vi "Set Node Action.vi"(8 "error in (no error)":errorcluster, 9 "action-only":bool, 10 "nodeIndex":i32, 11 "FSM in":refnum<class "FSM.Graph.lvclass">) -> (0 "error out":errorcluster, 3 "FSM out":refnum<class "FSM.Graph.lvclass">)   [LabVIEW 2015, in "FSM.Graph.lvclass"]
uses:
  FSM.Graph.lvclass
  FSM.Graph.lvclass/FSM.Graph.ctl
  FSM.Node/Shape.ctl
  FSM.Node/FSM.Node.lvclass/FSM.Node.ctl
  FSM.Node/Write Shape.vi
  FSM.Node/FSM.Node.lvclass
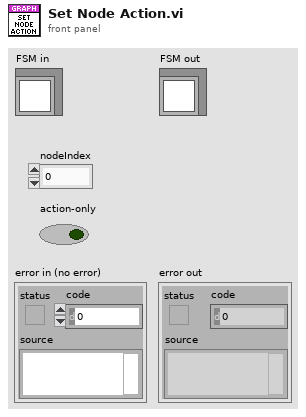
[diagram p1: front panel]
types:
  T1 = typedef "FSM.Node.lvclass/Shape.ctl" = enum16{"Default", "Start", "Action", "End"}
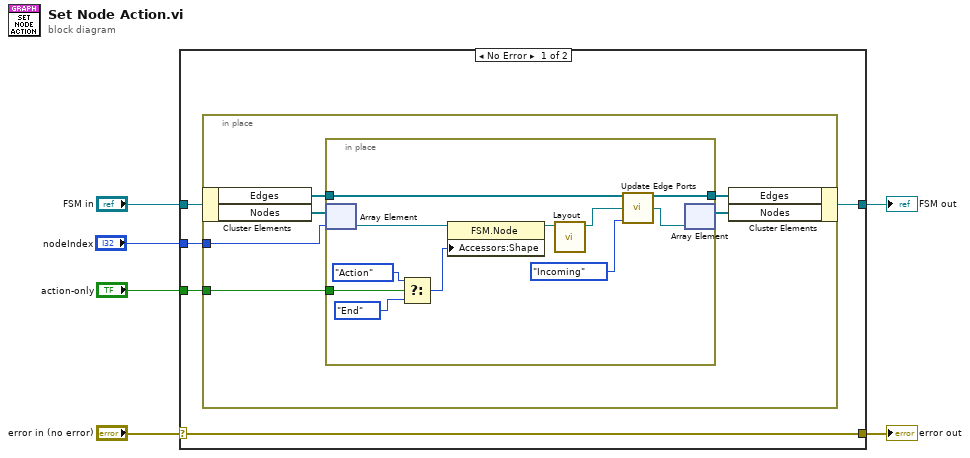
[diagram p0: block diagram]
diagram:
  n1 = case shown="No Error" "error in (no error)" {
    selector: "error in (no error)" -> [w11 w30]
    tunnel: [w11 w30] -> w5
    tunnel: [w8 w29] -> w3
    tunnel: "FSM in" -> [w10 w29]
    tunnel: "nodeIndex" -> [w9 _]
    tunnel: "action-only" -> [w7 _]
    frame No Error {
      n2 = in-place {
        in-place-border: w9 -> [w16]
        in-place-border: w7 -> [w12]
        n3 = in-place-cluster #1(w10) -> ("Edges"=w14:refnum<class "FSM.Edge.lvclass">[], "Nodes"=w17:refnum<class "FSM.Node.lvclass">[])
        n4 = in-place {
          in-place-border: w14 -> [w28]
          in-place-border: [w27] -> w13
          in-place-border: w12 -> [w23]
          n5 = in-place-array #2(w17, w16) -> (w25:refnum<class "FSM.Node.lvclass">)
          n6 = Select(t=Shape."Action", s=w23, f=Shape."End" ("Shape")) -> (s? t:f=w21:T1)
          n7 = property class="FSM.Node"(reference=w25, "Accessors:Shape"=w21) -> (reference out=w19:refnum<class "FSM.Node.lvclass">)  [unwired: 1 in, 1 out]
          n8 = call "Layout.vi"("FSM in"=w19) -> ("FSM out"=w18:refnum<class "FSM.Node.lvclass">)  [unwired: 9 in, 1 out]
          n9 = call "Update Edge Ports.vi"("Edges In"=w28, "FSM.Node In"=w18, "Edges"=enum16{"Incoming", "Outgoing"}."Incoming") -> ("Edges Out"=w27:refnum<class "FSM.Edge.lvclass">[], "FSM.Node thru"=w26:refnum<class "FSM.Node.lvclass">)  [unwired: 11 in]
          n10 = in-place-array #2(w26) -> (w15:refnum<class "FSM.Node.lvclass">[])  [unwired: 1 out]
        }
        n11 = in-place-cluster #1("Edges"=w13, "Nodes"=w15) -> (w8:refnum<class "FSM.Graph.lvclass">)
      }
    }
    frame Error {
    }
  }
  "error out" <- w5
  "FSM out" <- w3
